vi "Angle Aiming Mode.vi"(9 "Y Axis":dbl, 10 "Motor Scale":dbl, 11 "Vision Tracking Enable":bool) -> (3 "Motor Output":dbl)   [LabVIEW 2014]
uses:
  Robot Global Data.vi
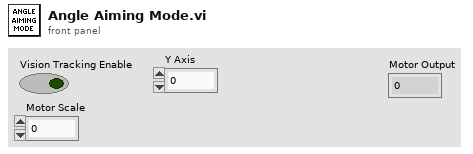
[diagram p1: front panel]
types:
  T1 = cluster{"Center Position":cluster{"X":dbl, "Y":dbl}, "Distance (ft)":dbl, "Center":bool}[]
  T2 = cluster{"Center Position":cluster{"X":dbl, "Y":dbl}, "Distance (ft)":dbl, "Center":bool}
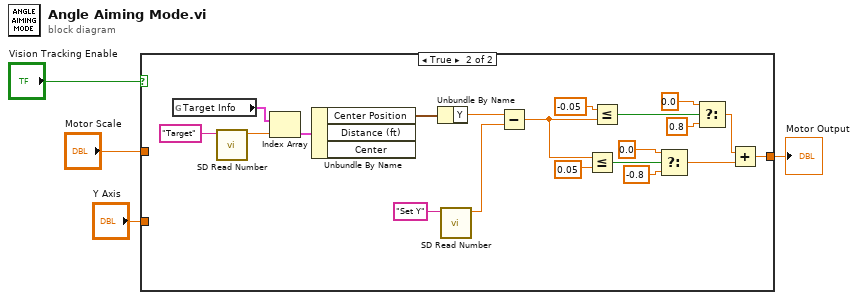
[diagram p0: block diagram]
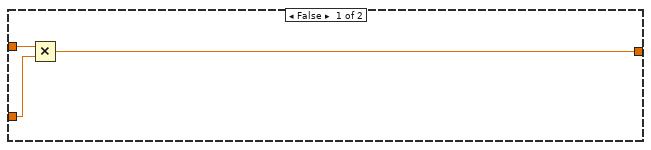
[diagram p2: hidden frame]
diagram:
  n1 = case shown="True" "Vision Tracking Enable" {
    tunnel: "Y Axis" -> [w7 _]
    tunnel: "Motor Scale" -> [w6 _]
    tunnel: [w5 w14] -> w1
    frame False {
      n2 = Multiply(x=w6, y=w7) -> (x*y=w5:dbl)
    }
    frame True {
      n3 = global read "Robot Global Data.vi" "Target Info"() -> (w12:T1)
      n4 = call <vilib>:"SD Read Number.vi"("Name"="Target" ("refnum name")) -> ("Numeric"=w9:dbl)  [unwired: 8 in, 2 out]
      n5 = Index Array(array=w12, index=w9) -> (element=w11:T2)
      n6 = Unbundle By Name(w11) -> ("Center Position"=w13:cluster{"X":dbl, "Y":dbl})  [unwired: 2 out]
      n7 = Unbundle By Name(w13) -> ("Y"=w8:dbl)
      n8 = call <vilib>:"SD Read Number.vi"("Name"="Set Y" ("refnum name")) -> ("Numeric"=w24:dbl)  [unwired: 8 in, 2 out]
      n9 = Subtract(x=w8, y=w24) -> (x-y=w23:dbl)
      n10 = Less Or Equal?(x=w23, y=0.05) -> (x <= y?=w21:bool)
      n11 = Less Or Equal?(x=-0.05, y=w23) -> (x <= y?=w22:bool)
      n12 = Select(t=0.0, s=w21, f=-0.8) -> (s? t:f=w15:dbl)
      n13 = Select(t=0.0, s=w22, f=0.8) -> (s? t:f=w16:dbl)
      n14 = Add(x=w16, y=w15) -> (x+y=w14:dbl)
    }
  }
  "Motor Output" <- w1
